vi "KMAX config read.vi"(11 "config file location":path) -> (0 "XScale.Minimum":dbl, 1 "Integration Time (5 ms)":dbl=0.25, 2 "Camera Name":refnum<k21> caption="IMAQdx Session", 4 "XScale.Maximum":dbl, 5 "configuration file path":path, 6 "Background":bool, 8 "Autoscale":bool)   [LabVIEW 2023]
uses:
  <vilib>/Utility/config.llb/Read Key (Double).vi
  <vilib>/Utility/config.llb/Read Key (String).vi
  <vilib>/Utility/config.llb/Read Key (Boolean).vi
  <vilib>/Utility/config.llb/NI_LVConfig.lvlib
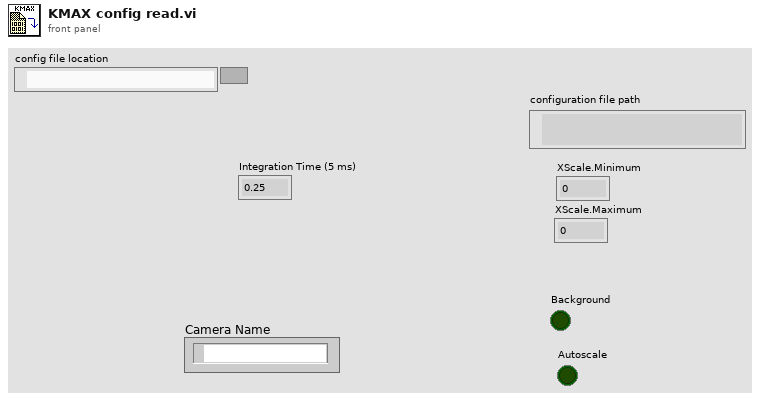
[diagram p1: front panel]
types:
  T1 = typedef "NI_LVConfig.lvlib/Config Data RefNum.ctl" = refnum<k1>
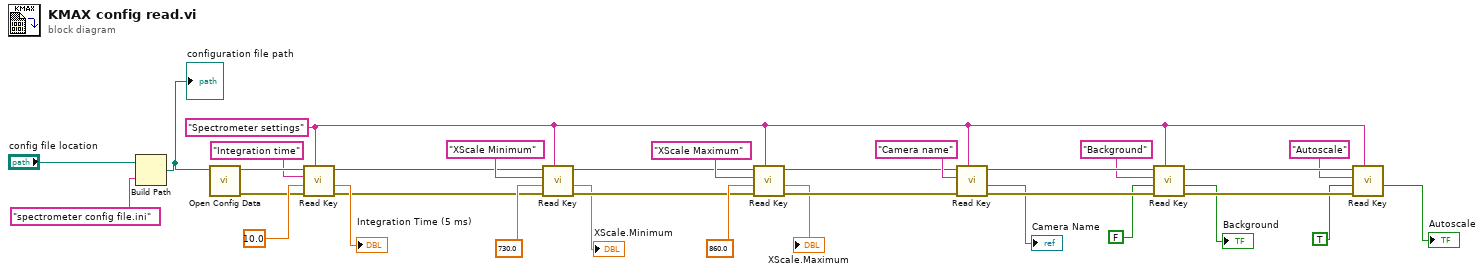
[diagram p0: block diagram]
diagram:
  w13 = "Spectrometer settings" ("section")
  n1 = Build Path(base path="config file location", name or relative path="spectrometer config file.ini") -> (appended path=w26:path)
  "configuration file path" <- w26
  n2 = call <vilib>:"Open Config Data.vi"("configuration file path"=w26) -> ("error out"=w28:errorcluster, "refnum"=w33:T1)  [unwired: 8 in, 1 out]
  n3 = call-poly <vilib>:"Read Key.vi"("section"=w13, "error in (no error)"=w28, "default value"=10.0, "key"="Integration time", "refnum"=w33) -> ("error out"=w18:errorcluster, "value"=→"Integration Time (5 ms)":dbl, "refnum out"=w21:T1)  [unwired: 3 in, 1 out]
  n4 = call-poly <vilib>:"Read Key.vi"("section"=w13, "error in (no error)"=w18, "default value"=730.0, "key"="XScale Minimum", "refnum"=w21) -> ("error out"=w17:errorcluster, "value"=→"XScale.Minimum":dbl, "refnum out"=w20:T1)  [unwired: 3 in, 1 out]
  n5 = call-poly <vilib>:"Read Key.vi"("section"=w13, "error in (no error)"=w17, "default value"=860.0, "key"="XScale Maximum", "refnum"=w20) -> ("error out"=w16:errorcluster, "value"=→"XScale.Maximum":dbl, "refnum out"=w19:T1)  [unwired: 3 in, 1 out]
  n6 = call-poly <vilib>:"Read Key.vi"("section"=w13, "error in (no error)"=w16, "key"="Camera name", "refnum"=w19) -> ("error out"=w10:errorcluster, "value"=→"Camera Name":string, "refnum out"=w12:T1)  [unwired: 4 in, 1 out]
  n7 = call-poly <vilib>:"Read Key.vi"("section"=w13, "error in (no error)"=w10, "default value"=FALSE, "key"="Background", "refnum"=w12) -> ("error out"=w9:errorcluster, "value"=→"Background":bool, "refnum out"=w11:T1)  [unwired: 3 in, 1 out]
  n8 = call-poly <vilib>:"Read Key.vi"("section"=w13, "error in (no error)"=w9, "default value"=TRUE, "key"="Autoscale", "refnum"=w11) -> ("value"=→"Autoscale":bool)  [unwired: 3 in, 3 out]
